vi "Charger_Multi-Channel Execute.vi"(6 "STOP Refnum":refnum<vi>, 7 "Status Refnum  Array":T1[](array[typedef]), 8 "error in":errorcluster) -> (0 "error out":errorcluster)   [LabVIEW 2020]
doc: "This function performs the following:\n\n1) Creates a single semaphore reference.\n2) Runs all six charger positions in parallel with semaphore arbitration.\n3) Deletes the semaphore reference."
uses:
  Charger_Status Refnum.ctl
  Drivers/Charger Test Set/Charger_Input Control.ctl
panel:
  out "error out 6":errorcluster
  out "error out 5":errorcluster
  out "error out 4":errorcluster
  out "error out 3":errorcluster
  out "error out 2":errorcluster
  out "error out 1":errorcluster
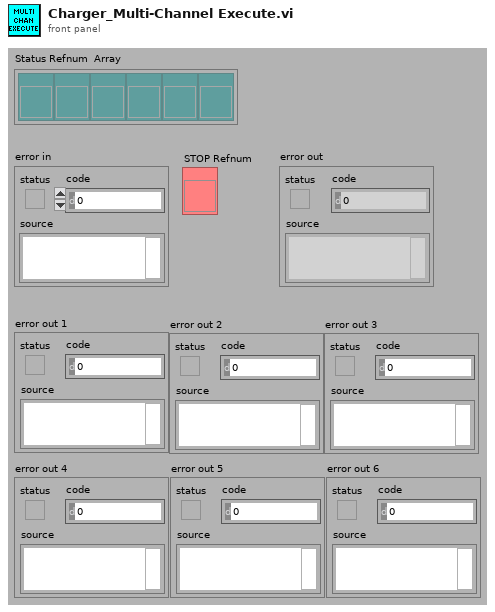
[diagram p1: front panel]
types:
  T1 = typedef "Charger_Status Refnum.ctl" = refnum<vi>
  T2 = typedef "Semaphore RefNum" = refnum<k1>
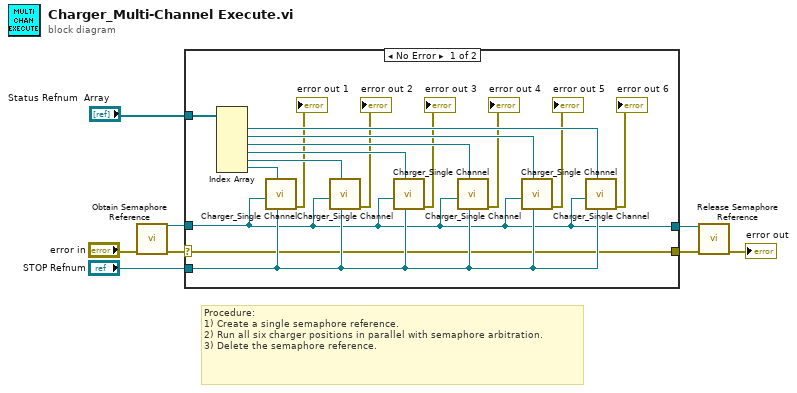
[diagram p0: block diagram]
diagram:
  # "Procedure:\n1) Create a single semaphore reference.\n2) Run all six charger positions in parallel with semaphore arbitration.\n3) Delete the semaphore reference."
  n1 = call <vilib>:"Obtain Semaphore Reference.vi"("error in (no error)"="error in") -> ("error out"=w3:errorcluster, "semaphore"=w2:T2)  [unwired: 4 in, 1 out]
  n2 = case shown="No Error" w3 {
    selector: w3 -> [w9 w26]
    tunnel: [w9 w26] -> w5
    tunnel: "Status Refnum  Array" -> [w23 _]
    tunnel: "STOP Refnum" -> [w18 _]
    tunnel: [w10 w25] -> w4
    tunnel: w2 -> [w10 w25]
    frame No Error {
      n3 = Index Array(array=w23) -> (element #1=w24:T1, element #2=w22:T1, element #3=w21:T1, element #4=w20:T1, element #5=w19:T1, element #6=w17:T1)  [unwired: 6 in]
      n4 = call "Charger_Single Channel.vi"("Stop Refnum"=w18, "Status Refnum"=w17, "semaphore"=w10) -> ("error out"=→"error out 1":errorcluster)  [unwired: 8 in]
      n5 = call "Charger_Single Channel.vi"("Stop Refnum"=w18, "Status Refnum"=w19, "semaphore"=w10) -> ("error out"=→"error out 2":errorcluster)  [unwired: 8 in]
      n6 = call "Charger_Single Channel.vi"("Stop Refnum"=w18, "Status Refnum"=w20, "semaphore"=w10) -> ("error out"=→"error out 3":errorcluster)  [unwired: 8 in]
      n7 = call "Charger_Single Channel.vi"("Stop Refnum"=w18, "Status Refnum"=w21, "semaphore"=w10) -> ("error out"=→"error out 4":errorcluster)  [unwired: 8 in]
      n8 = call "Charger_Single Channel.vi"("Stop Refnum"=w18, "Status Refnum"=w22, "semaphore"=w10) -> ("error out"=→"error out 5":errorcluster)  [unwired: 8 in]
      n9 = call "Charger_Single Channel.vi"("Stop Refnum"=w18, "Status Refnum"=w24, "semaphore"=w10) -> ("error out"=→"error out 6":errorcluster)  [unwired: 8 in]
    }
    frame Error {
    }
  }
  n10 = call <vilib>:"Release Semaphore Reference.vi"("error in (no error)"=w5, "semaphore"=w4) -> ("error out"=→"error out":errorcluster)  [unwired: 8 in, 1 out]
